vi "SlashCodes.vi"() -> ()   [LabVIEW 2019]
panel:
  in  "Hardware":string
  out "ReceivedHWData":string
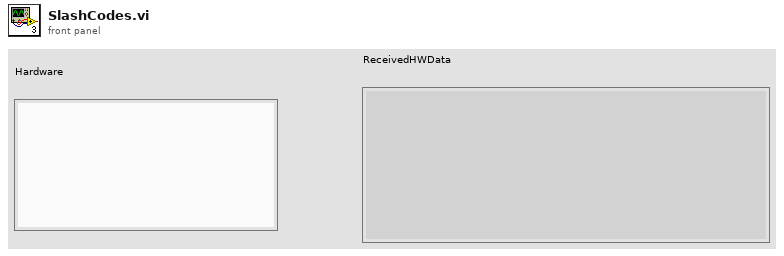
[diagram p1: front panel]
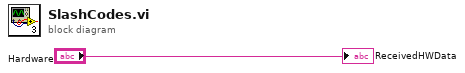
[diagram p0: block diagram]
diagram:
  "ReceivedHWData" <- "Hardware"
